vi "Get User and Language.vi"(8 "错误输入（无错误）":errorcluster) -> (0 "错误输出":errorcluster, 2 "应用程序:语言":string, 3 "应用程序:用户名":string)   [LabVIEW 2012, in "Application.lvlib"]
uses:
  Application.lvlib
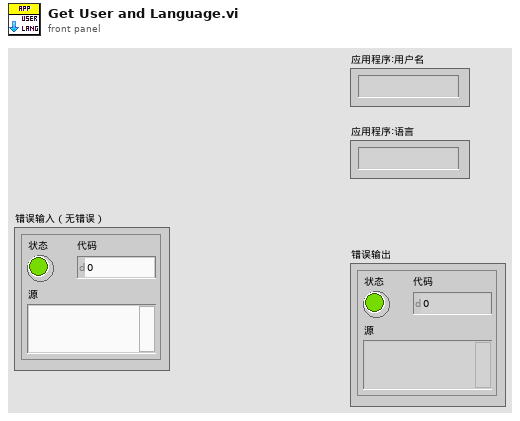
[diagram p1: front panel]
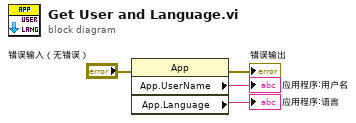
[diagram p0: block diagram]
diagram:
  n1 = property class="App"(error in="错误输入（无错误）") -> (error out=→"错误输出":errorcluster, "App.UserName"=→"应用程序:用户名":string, "App.Language"=→"应用程序:语言":string)  [unwired: 1 in, 1 out]
